vi "OFDM-SIM误比特率.vi"(2 "比特数":i32=25000, 3 "输出比特":i8[](array[numeric]), 4 "输入比特":i8[](array[numeric])) -> (0 "误比特率":dbl, 1 "错误个数":dbl)   [LabVIEW 2018]
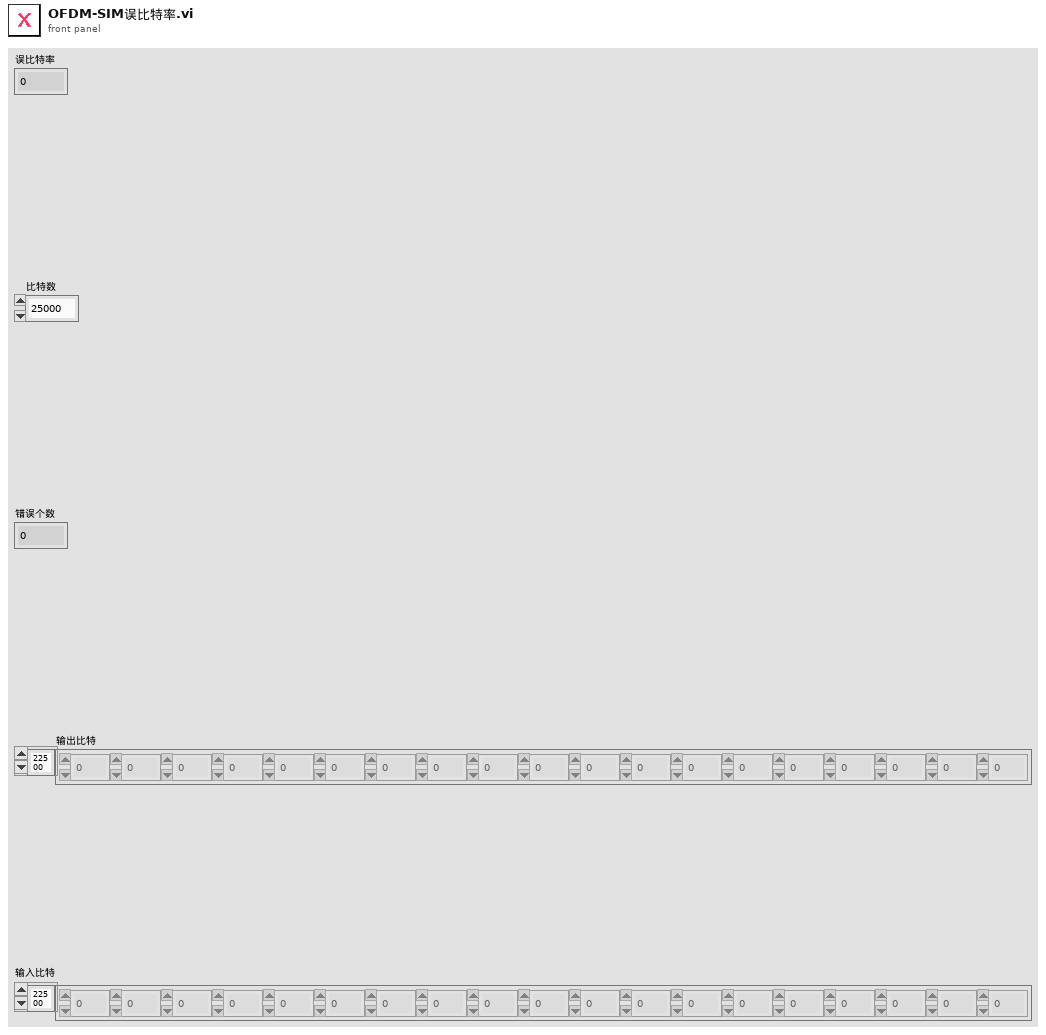
[diagram p1: front panel]
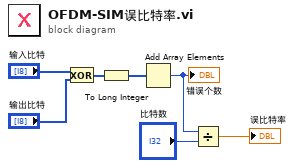
[diagram p0: block diagram]
diagram:
  n1 = Exclusive Or(1:"输出比特", 2:"输入比特") -> (0:w7:i8[])
  n2 = To Long Integer(number=w7) -> (32bit integer=w6:i32[])
  n3 = Add Array Elements(numeric array=w6) -> (sum=w4:i32)
  "错误个数" <- w4
  n4 = Divide(x=w4, y="比特数") -> (x/y=→"误比特率":dbl)
